vi "Create DigiPattern File.vi"(8 "error in (no error)":errorcluster, 9 "Pattern Name":string, 10 "BML Frame Array":refnum<class "BML_Frame_Root.lvclass">[](array[class]), 11 "BML_DigiPattern_Generator.lvclass":refnum<class "BML_DigiPattern_Generator.lvclass">) -> (0 "error out":errorcluster, 3 "BML_DigiPattern_Generator.lvclass out":refnum<class "BML_DigiPattern_Generator.lvclass">)   [LabVIEW 2016, in "BML_DigiPattern_Generator.lvclass"]
uses:
  BML_DigiPattern_Generator.lvclass
  BML_Frame_Root/BML_Frame_Root.lvclass
  BML_DigiPattern_Generator.lvclass/BML_DigiPattern_Generator.ctl
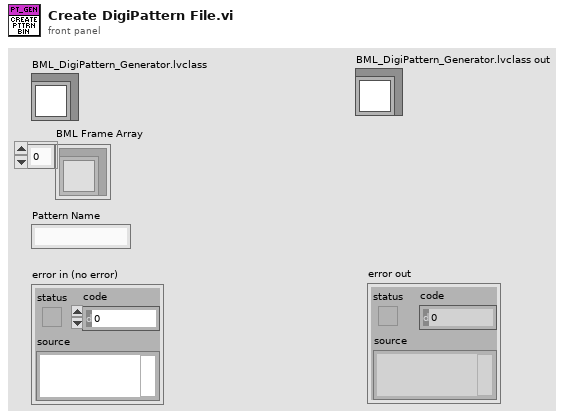
[diagram p1: front panel]
types:
  T1 = enum16{"open", "replace", "create", "open or create", "replace or create", "replace or create with confirmation"}
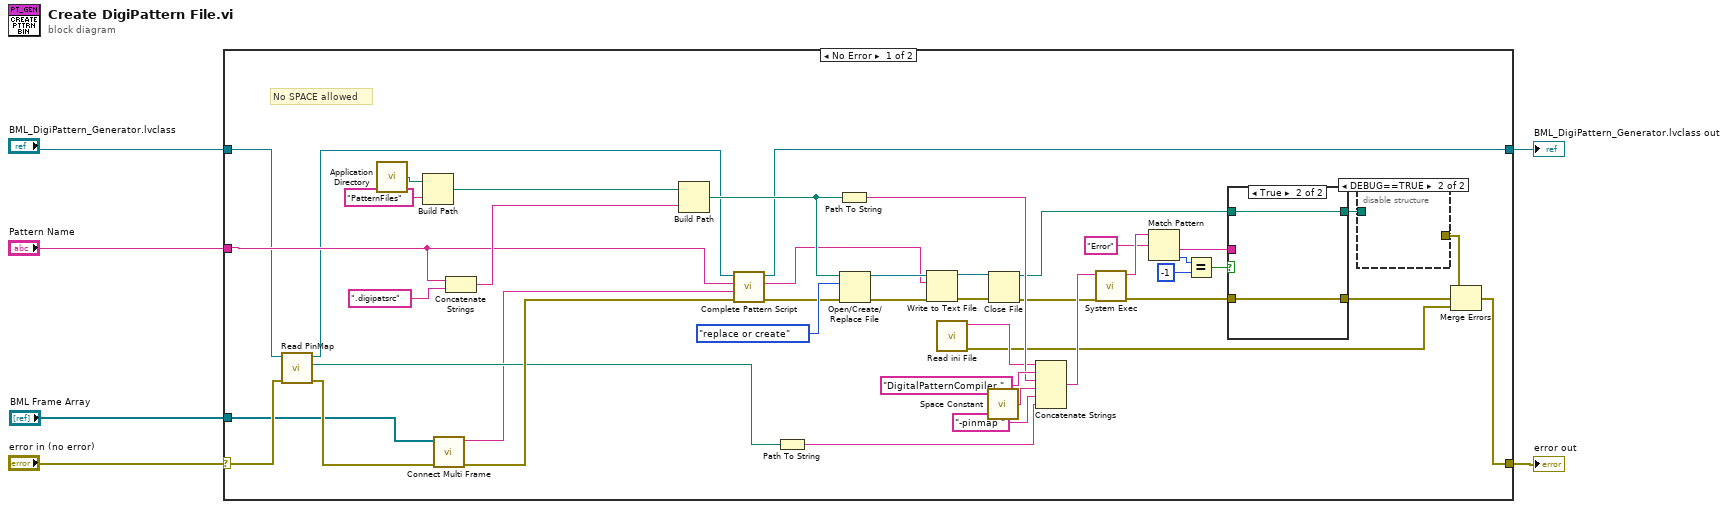
[diagram p0: block diagram]
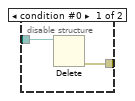
[diagram p2: hidden frame]
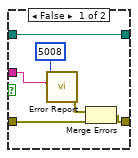
[diagram p3: hidden frame]
diagram:
  n1 = case shown="No Error" "error in (no error)" {
    selector: "error in (no error)" -> [w11 w62]
    tunnel: [w30 w62] -> w5
    tunnel: [w19 w61] -> w2
    tunnel: "BML_DigiPattern_Generator.lvclass" -> [w13 w61]
    tunnel: "Pattern Name" -> [w18 _]
    tunnel: "BML Frame Array" -> [w9 _]
    frame No Error {
      # "No SPACE allowed"
      n2 = call "Read PinMap.vi"("error in (no error)"=w11, "BML_DigiPattern_Generator in"=w13) -> ("error out"=w10:errorcluster, "PinMap"=w8:path, "BML_DigiPattern_Generator out"=w12:refnum<class "BML_DigiPattern_Generator.lvclass">)  [unwired: 7 in]
      n3 = call <vilib>:"Application Directory.vi"() -> ("Application Directory"=w26:path)
      n4 = Build Path(base path=w26, name or relative path="PatternFiles") -> (appended path=w24:path)
      n5 = call "Connect Multi Frame.vi"("error in (no error)"=w10, "BML Frame Array"=w9) -> ("error out"=w14:errorcluster, "Connected Frame Contents"=w7:string)  [unwired: 8 in]
      n6 = Concatenate Strings(w18, ".digipatsrc" ("string")) -> (w49:string)
      n7 = Build Path(base path=w24, name or relative path=w49) -> (appended path=w44:path)
      n8 = call "Complete Pattern Script.vi"("error in (no error)"=w14, "Pattern Contents"=w7, "Pattern Name"=w18, "BML_DigiPattern_Generator.lvclass"=w12) -> ("error out"=w20:errorcluster, "All Pattern Script out"=w17:string, "BML_DigiPattern_Generator.lvclass out"=w19:refnum<class "BML_DigiPattern_Generator.lvclass">)  [unwired: 5 in]
      n9 = Path To String(path=w8) -> (string=w40:string)
      n10 = Path To String(path=w44) -> (string=w43:string)
      n11 = Open/Create/Replace File(file path (use dialog)=w44, error in=w20, operation (0:open)=T1."replace or create") -> (refnum out=w47:refnum<file>, error out=w46:errorcluster)  [unwired: 3 in, 1 out]
      n12 = Write to Text File(file (use dialog)=w47, text=w17, error in=w46) -> (refnum out=w29:refnum<file>, error out=w28:errorcluster)  [unwired: 1 in, 1 out]
      n13 = call "Read ini File.vi"() -> ("error out"=w15:errorcluster, "value"=w16:string)  [unwired: 10 in]
      n14 = call <vilib>:"Space Constant.vi"() -> ("String"=w42:string)
      n15 = Close File(refnum=w29, error in=w28) -> (path=w22:path, error out=w27:errorcluster)
      n16 = Concatenate Strings(w16, "DigitalPatternCompiler " ("string"), w43, w42, "-pinmap " ("string"), w40) -> (w39:string)
      n17 = call <vilib>:"System Exec.vi"("error in (no error)"=w27, "command line"=w39) -> ("error out"=w32:errorcluster, "standard output"=w38:string)  [unwired: 6 in, 2 out]
      n18 = Match Pattern(string=w38, regular expression="Error") -> (after substring=w33:string, offset past match=w36:i32)  [unwired: 1 in, 2 out]
      n19 = Equal?(x=w36, y=-1) -> (x = y?=w34:bool)
      n20 = case shown="True" w34 {
        tunnel: w33 -> [w54 _]
        tunnel: w32 -> [w58 w60]
        tunnel: [w57 w60] -> w31
        tunnel: w22 -> [w56 w59]
        tunnel: [w56 w59] -> w21
        frame False {
          n21 = call "Error Report.vi"("Additional info"=w54, "Error Code"=i16 5008) -> ("error out"=w53:errorcluster)  [unwired: 9 in]
          n22 = Merge Errors(w53, w58) -> (w57:errorcluster)
        }
        frame True {
        }
      }
      n23 = disable-structure shown="DEBUG==TRUE" {
        disable-tunnel: [w52 _] -> w23
        disable-tunnel: w21 -> [w51 _]
        frame condition #0 {
          n24 = Delete(path (use dialog)=w51) -> (error out=w52:errorcluster)  [unwired: 4 in, 2 out]
        }
        frame condition #1 (active) {
        }
      }
      n25 = Merge Errors(w23, w31, w15) -> (w30:errorcluster)
    }
    frame Error {
    }
  }
  "error out" <- w5
  "BML_DigiPattern_Generator.lvclass out" <- w2
